vi "IEEE754format.vi"(10 "Number":sgl=-101.101 format="%.12f", 11 "Hex String In":string) -> (2 "Number":sgl=92.92 format="%.10f", 3 "hex integer string":string)   [LabVIEW 2014]
doc: "This VI shows how LabVIEW stores SGL floating-point numbers in memory in binary format. The 32-bit binary number is based on the following IEEE 754 format:\n\n1 bit for the SIGN\n8 bits for the EXPONENT\n23 bits for the MANTISSA\n\nThe formula for the conversion is the following:\n\nSGL = (-1)^SIGN * 1.MANTISSA * 2^(EXPONENT-127)\n\nYou can use this VI to convert SGL numbers to their binary storage equivalent, and vice versa."
panel:
  out "Byte Array Out":bool[](array[boolean])
  out "Sign":bool=TRUE
  out "Mantissa":bool[](array[boolean])=[TRUE, FALSE, FALSE, TRUE, FALSE, TRUE, FALSE, FALSE, FALSE, TRUE, TRUE, FALSE, FALSE, TRUE, TRUE, TRUE, FALSE, TRUE, TRUE, FALSE, TRUE, TRUE, FALSE]
  out "Exponent":bool[](array[boolean])=[TRUE, FALSE, FALSE, FALSE, FALSE, TRUE, FALSE, TRUE]
  out "Exponent":sgl=6.0 format="%.2f"
  out "Mantissa":sgl=1.5797031 format="%.8f"
  out "Exponent":i32=6
  out "Mantissa":dbl=1.4518749713897705 format="%.8f"
  # "SGL to Binary Storage Format"
  # "Enter Decimal Number -->"
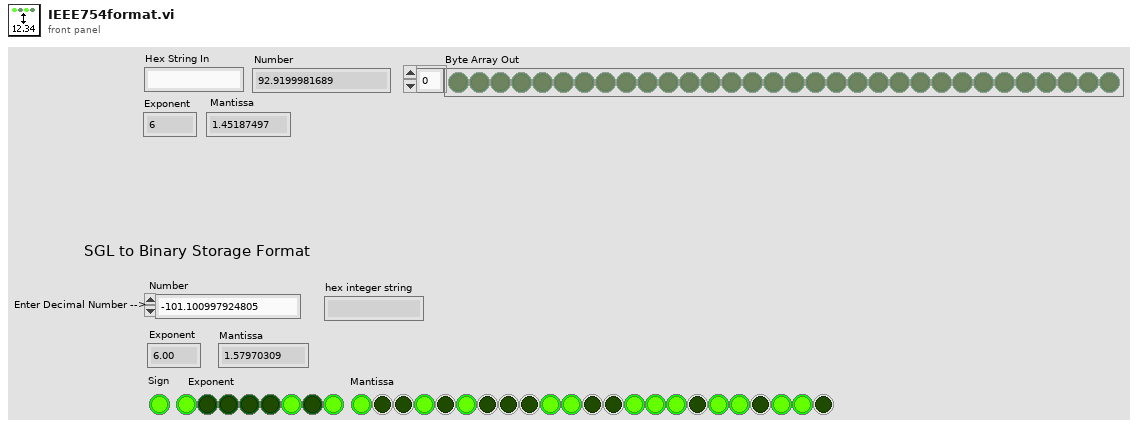
[diagram p1: front panel]
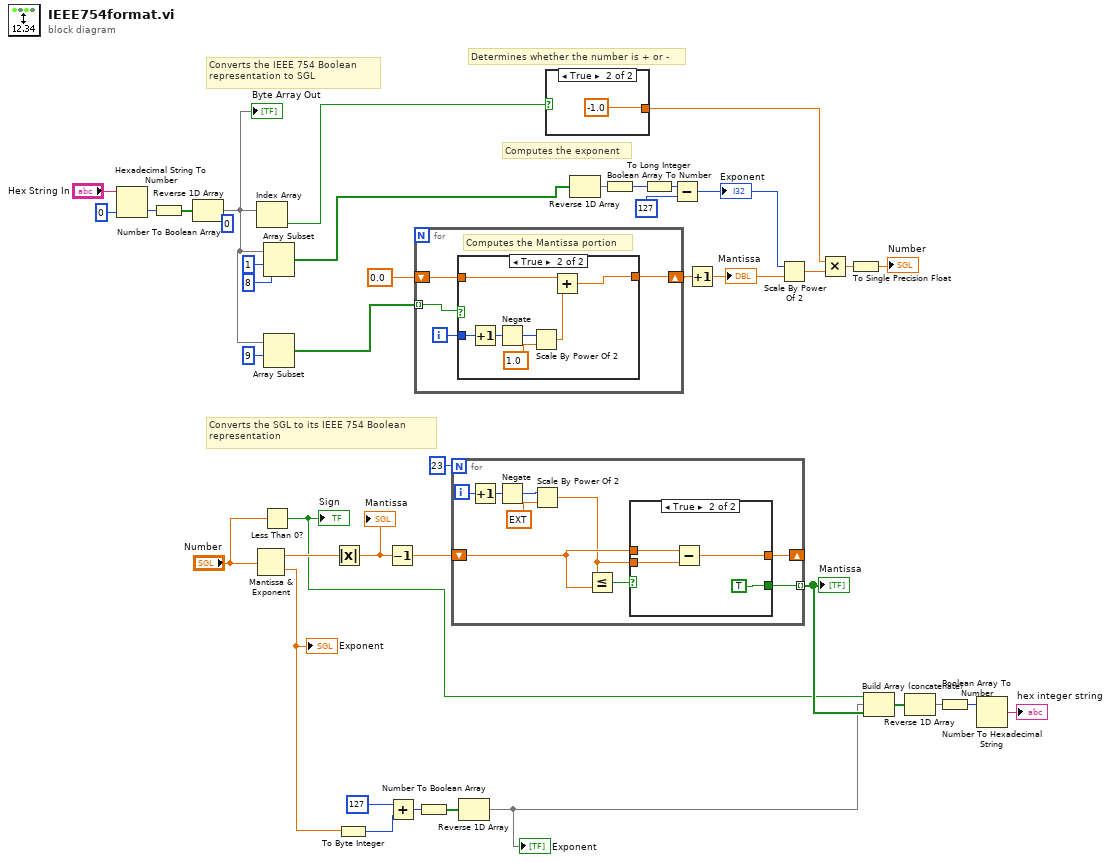
[diagram p0: block diagram]
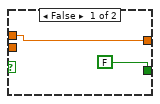
[diagram p2: hidden frame]
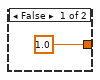
[diagram p3: hidden frame]
diagram:
  (unwired) 0 ("index")
  # "Converts the SGL to its IEEE 754 Boolean \nrepresentation"
  # "Converts the IEEE 754 Boolean \nrepresentation to SGL"
  # "Computes the exponent"
  # "Determines whether the number is + or -"
  n1 = Hexadecimal String To Number(string="Hex String In", default (0uL)=u32 0 ("default (0 U32)")) -> (number=w9:u32)  [unwired: 1 in, 1 out]
  n2 = Number To Boolean Array(number=w9) -> (Boolean array=w8:bool[])
  n3 = Reverse 1D Array(array=w8) -> (reversed array=w3:bool[])
  "Byte Array Out" <- w3
  n4 = Mantissa & Exponent(0:"Number") -> (1:w20:sgl, 2:w23:sgl)
  "Exponent" <- w23
  n5 = Index Array(array=w3) -> (element=w7:bool)  [unwired: 1 in]
  n6 = Less Than 0?(x="Number") -> (x < 0?=w16:bool)
  "Sign" <- w16
  n7 = Array Subset(array=w3, index=1, length=8) -> (w4:bool[])
  n8 = Array Subset(array=w3, index=9) -> (w1:bool[])  [unwired: 1 in]
  n9 = Absolute Value(x=w20) -> (abs(x)=w21:sgl)
  "Mantissa" <- w21
  n10 = To Byte Integer(number=w23) -> (8bit integer=w29:i8)
  n11 = Decrement(x=w21) -> (x-1=w25:sgl)
  n12 = Add(x=i8 127, y=w29) -> (x+y=w28:i8)
  n13 = for {
    tunnel: w1 -> [w44] mode=indexing
    shift-right: [w41] -> w39
    shift-left: 0.0 -> [w42]
    i -> [w43]
    # "Computes the Mantissa portion"
    n14 = case shown="True" w44 {
      tunnel: w43 -> [_ w52]
      tunnel: w42 -> [w45 w48]
      tunnel: [w45 w46] -> w41
      frame False {
      }
      frame True {
        n15 = Increment(x=w52) -> (x+1=w51:i32)
        n16 = Negate(x=w51) -> (-x=w50:i32)
        n17 = Scale By Power Of 2(n=w50, x=1.0) -> (x*2^n=w47:dbl)
        n18 = Add(x=w48, y=w47) -> (x+y=w46:dbl)
      }
    }
  }
  n19 = Number To Boolean Array(number=w28) -> (Boolean array=w27:bool[])
  n20 = for {
    N: 23 -> [_]
    shift-right: [w54] -> _
    shift-left: w25 -> [w56]
    tunnel: [w53] -> w18 mode=indexing
    i -> [w61]
    n21 = Increment(x=w61) -> (x+1=w60:i32)
    n22 = Negate(x=w60) -> (-x=w59:i32)
    n23 = Scale By Power Of 2(n=w59, x=ext 1.0) -> (x*2^n=w55:ext)
    n24 = Less Or Equal?(x=w55, y=w56) -> (x <= y?=w57:bool)
    n25 = case shown="True" w57 {
      tunnel: w56 -> [w62 w67]
      tunnel: w55 -> [_ w64]
      tunnel: [w62 w66] -> w54
      tunnel: [FALSE TRUE] -> w53
      frame False {
      }
      frame True {
        n26 = Subtract(x=w67, y=w64) -> (x-y=w66:ext)
      }
    }
  }
  "Mantissa" <- w18
  n27 = Reverse 1D Array(array=w27) -> (reversed array=w17:bool[])
  "Exponent" <- w17
  n28 = case shown="True" w7 {
    tunnel: [1.0 -1.0] -> w33
    frame False {
    }
    frame True {
    }
  }
  n29 = Reverse 1D Array(array=w4) -> (reversed array=w35:bool[])
  n30 = Boolean Array To Number(Boolean array=w35) -> (number=w31:u32)
  n31 = To Long Integer(number=w31) -> (32bit integer=w30:i32)
  n32 = Subtract(x=w30, y=127) -> (x-y=w32:i32)
  "Exponent" <- w32
  n33 = Increment(x=w39) -> (x+1=w37:dbl)
  "Mantissa" <- w37
  n34 = Scale By Power Of 2(n=w32, x=w37) -> (x*2^n=w36:dbl)
  n35 = Multiply(x=w33, y=w36) -> (x*y=w34:dbl)
  n36 = To Single Precision Float(number=w34) -> (single precision float=→"Number":sgl)
  n37 = Build Array (concatenate)(w16, w17, w18) -> (w13:bool[])
  n38 = Reverse 1D Array(array=w13) -> (reversed array=w12:bool[])
  n39 = Boolean Array To Number(Boolean array=w12) -> (number=w15:u32)
  n40 = Number To Hexadecimal String(2:w15) -> (0:→"hex integer string":string)  [unwired: 1 in]
